vi "Allocate Image.vi"(8 "Error In":errorcluster, 10 "Image Parameters":T4={"Channel Order"=enum."CL_LUMINANCE (Grayscale)", "Dimension"={"Depth"=1, "Height"=1, "Width"=1}, "Data Type"=enum."32f", "Offset"={"X"=1, "Y"=1, "Z"=1}} {"Dimension"."Width" min=1; "Dimension"."Height" min=1; "Dimension"."Depth" min=1}, 11 "Labview Device":T2) -> (0 "Error Out":errorcluster, 2 "Image Parameters Out":T4={"Channel Order"=enum."CL_LUMINANCE (Grayscale)", "Dimension"={"Depth"=1, "Height"=1, "Width"=1}, "Data Type"=enum."32f", "Offset"={"X"=1, "Y"=1, "Z"=1}} {"Dimension"."Width" min=1; "Dimension"."Height" min=1; "Dimension"."Depth" min=1}, 3 "Image Object":T1={"Device ID"=0, "Memeroy ID"=0, "Image Parameters"={"Channel Order"=enum."CL_LUMINANCE (Grayscale)", "Dimension"={"Depth"=1, "Height"=1, "Width"=1}, "Data Type"=enum."32f", "Offset"={"X"=0, "Y"=0, "Z"=0}}} {"Image Parameters"."Dimension"."Width" min=1; "Image Parameters"."Dimension"."Height" min=1; "Image Parameters"."Dimension"."Depth" min=1})   [LabVIEW 2012]
doc: "Allocates a 2D or 3D image based on the input parameters."
uses:
  Non-User VIs/Controls/Image Parameters.ctl
  Non-User VIs/Images/Channel Order.ctl
  User Controls/Array Dimensions.ctl
  Non-User VIs/Images/Data Type.ctl
  User Controls/Offset.ctl
  Non-User VIs/Controls/Device ID.ctl
  Non-User VIs/Controls/Image Object.ctl
  Non-User VIs/Controls/Memory ID.ctl
  Non-User VIs/Error Checking/Add Error Functional Global.vi
  OpenCLV x64.lvlib
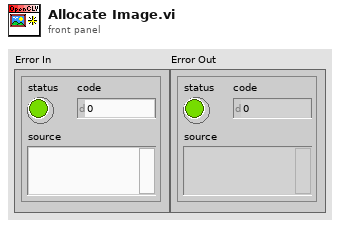
[diagram p1: front panel]
types:
  T1 = typedef "OpenCLV x64.lvlib/Image Object.ctl" = cluster{"Device ID":T2, "Memeroy ID":T3, "Image Parameters":T4}
  T2 = typedef "OpenCLV x64.lvlib/Device ID.ctl" = u64
  T3 = typedef "OpenCLV x64.lvlib/Memory ID.ctl" = u64
  T4 = typedef "OpenCLV x64.lvlib/Image Parameters.ctl" = cluster{"Channel Order":T5, "Dimension":T6, "Data Type":T7, "Offset":T8}
  T5 = typedef "OpenCLV x64.lvlib/Channel Order.ctl" = enum16{"CL_LUMINANCE (Grayscale)", "CL_INTENSITY (Opacity)", "CL_RGBA", "CL_ARGB", "CL_BGRA", "CL_RG", "CL_RA", "CL_R", "CL_A"}
  T6 = typedef "Array Dimensions.ctl" = cluster{"Depth":u64, "Height":u64, "Width":u64}
  T7 = typedef "OpenCLV x64.lvlib/Data Type.ctl" = enum16{"32f", "u8", "u16", "u32", "i8", "i16", "i32"}
  T8 = typedef "Offset.ctl" = cluster{"X":u64, "Y":u64, "Z":u64}
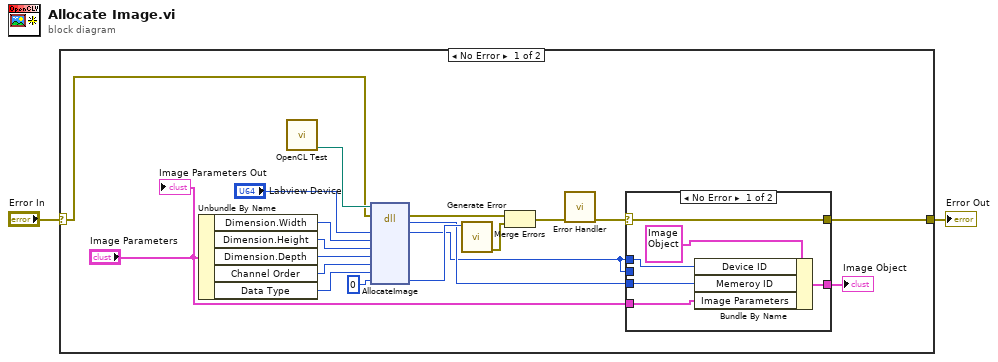
[diagram p0: block diagram]
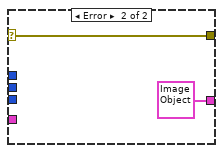
[diagram p2: hidden frame]
diagram:
  n1 = case shown="No Error" "Error In" {
    selector: "Error In" -> [w3 w30]
    tunnel: [w11 w30] -> w1
    frame No Error {
      n2 = Unbundle By Name("Image Parameters") -> ("Dimension.Width"=w13:u64, "Dimension.Height"=w14:u64, "Dimension.Depth"=w15:u64, "Channel Order"=w16:T5, "Data Type"=w17:T7)
      n3 = call "OpenCL Test.vi"() -> ("DLL To Use"=w7:path)  [unwired: 11 in]
      n4 = dll-call lib="C:/Users/bme-amcelroy-la/Desktop/OpenCLV/trunk/OpenCLV_x64_1.0/OpenCLV_x64.dll" fn="AllocateImage"(path in=w7, error in=w3, "Labview Device"="Labview Device", "Width"=w13, "Height"=w14, "Depth"=w15, "Channel Order"=w16, "Data Type"=w17, "Error"=0) -> (error out=w19:errorcluster, "return type"=w10:u64, "Labview Device"=w9:u64, "Error"=w21:i32)  [unwired: 6 in, 1 out]
      n5 = call "Generate Error.vi"("Error"=w21) -> ("error out"=w20:errorcluster)  [unwired: 10 in]
      n6 = Merge Errors(w19, w20) -> (w5:errorcluster)
      n7 = call-poly "Error Handler.vi"("Error In"=w5) -> ("Error Out"=w4:errorcluster)  [unwired: 10 in]
      n8 = case shown="No Error" w4 {
        selector: w4 -> [w23 w29]
        tunnel: [w23 w29] -> w11
        tunnel: w10 -> [w24 _]
        tunnel: w9 -> [w27 _]
        tunnel: w9 -> [_ _]
        tunnel: "Image Parameters" -> [w25 _]
        tunnel: [w22 T1 {"Device ID"=0, "Memeroy ID"=0, "Image Parameters"={"Channel Order"=enum."CL_LUMINANCE (Grayscale)", "Dimension"={"Depth"=1, "Height"=1, "Width"=1}, "Data Type"=enum."32f", "Offset"={"X"=0, "Y"=0, "Z"=0}}} ("Memory Object")] -> w6
        frame No Error {
          n9 = Bundle By Name(cluster=T1 {"Device ID"=0, "Memeroy ID"=0, "Image Parameters"={"Channel Order"=enum."CL_LUMINANCE (Grayscale)", "Dimension"={"Depth"=0, "Height"=0, "Width"=0}, "Data Type"=enum."32f", "Offset"={"X"=0, "Y"=0, "Z"=0}}} ("Memory Object"), "Device ID"=w27, "Memeroy ID"=w24, "Image Parameters"=w25) -> (w22:T1)
        }
        frame Error {
        }
      }
      "Image Object" <- w6
      "Image Parameters Out" <- "Image Parameters"
    }
    frame Error {
    }
  }
  "Error Out" <- w1
